vi "Get Variables.vi"(8 "error in (no error)":errorcluster, 11 "Bitwise Operations in":refnum<class "Bitwise Functions.lvclass">) -> (0 "error out":errorcluster, 2 "Variables":variant, 3 "Bitwise Operations out":refnum<class "Bitwise Functions.lvclass">)   [LabVIEW 2016, in "Bitwise Functions.lvclass"]
uses:
  Bitwise Functions.lvclass
  Bitwise Functions.lvclass/Bitwise Functions.ctl
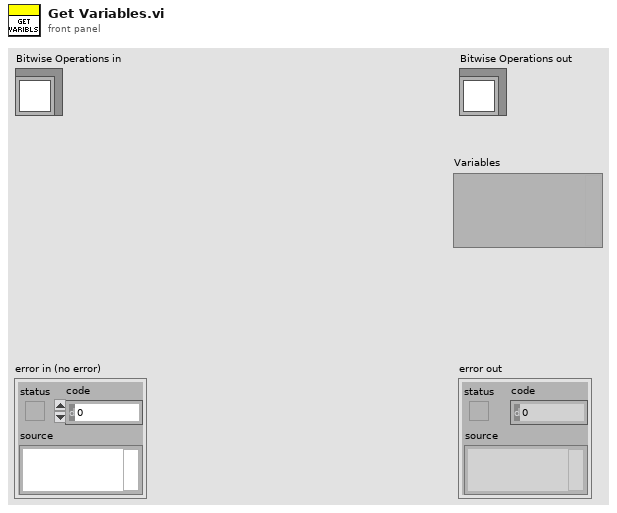
[diagram p1: front panel]
types:
  T1 = typedef "Bitwise Functions.lvclass/Variables.ctl" = cluster{"Var1":i32, "Var2":i32}
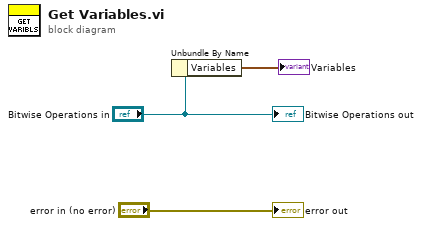
[diagram p0: block diagram]
diagram:
  n1 = Unbundle By Name("Bitwise Operations in") -> ("Variables"=→"Variables":T1)
  "error out" <- "error in (no error)"
  "Bitwise Operations out" <- "Bitwise Operations in"
